vi "Property Finder (SubVI).vi"(8 "error in (no error)":errorcluster, 10 "Enum":enum16{"Read File", "Search for Property Name"}(ring), 11 "Property Name":string) -> (0 "error out":errorcluster, 3 "Property Value":string)   [LabVIEW 2018]
uses:
  <vilib>/regexp/Match Regular Expression.xnode
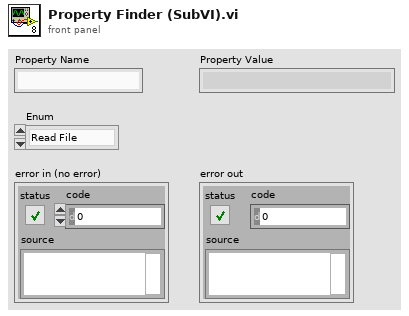
[diagram p1: front panel]
types:
  T1 = enum16{"open", "replace", "create", "open or create", "replace or create", "replace or create with confirmation"}
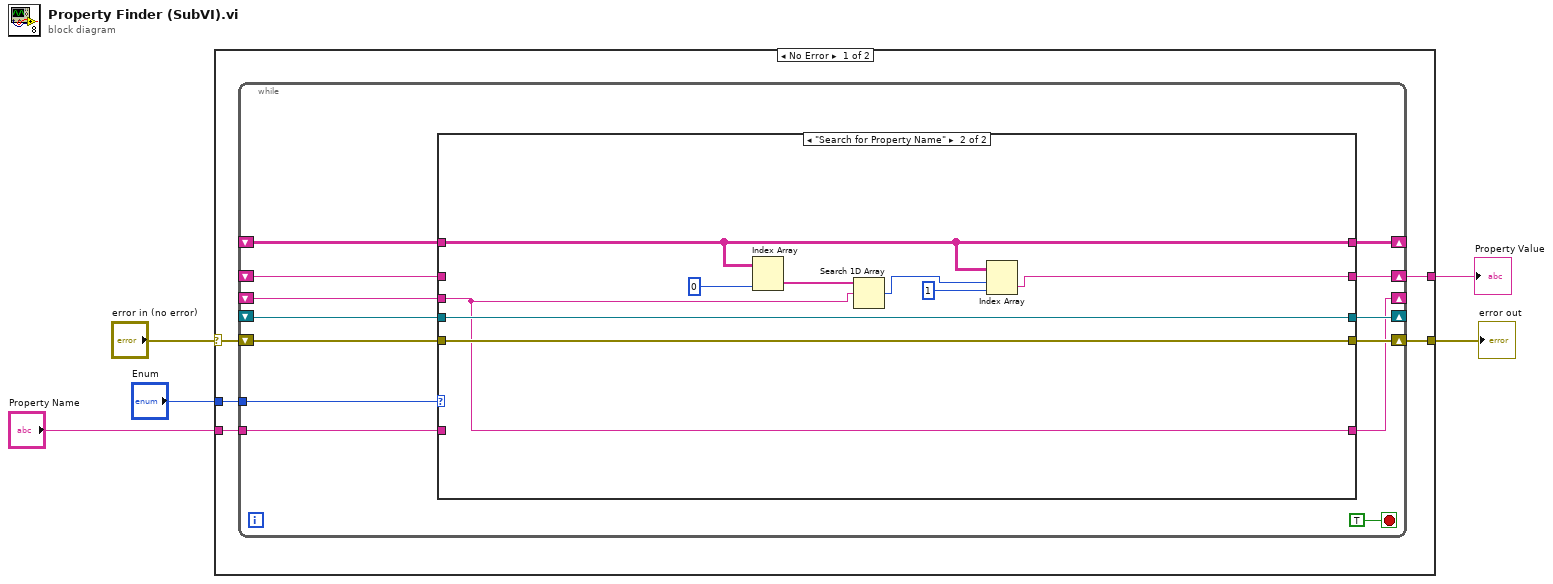
[diagram p0: block diagram]
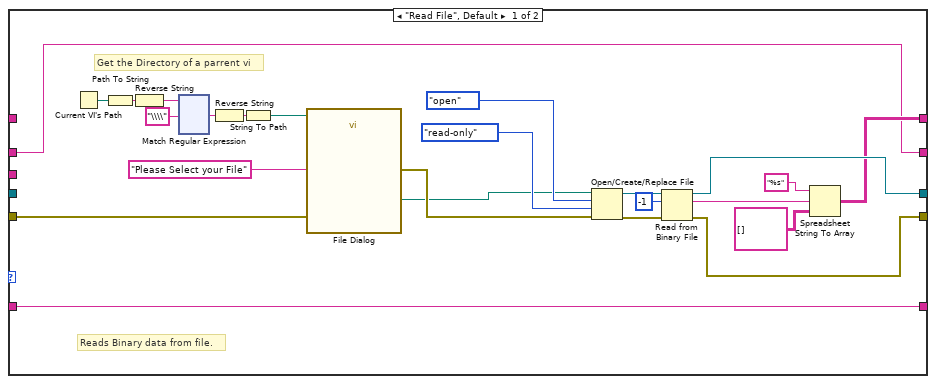
[diagram p2: hidden frame]
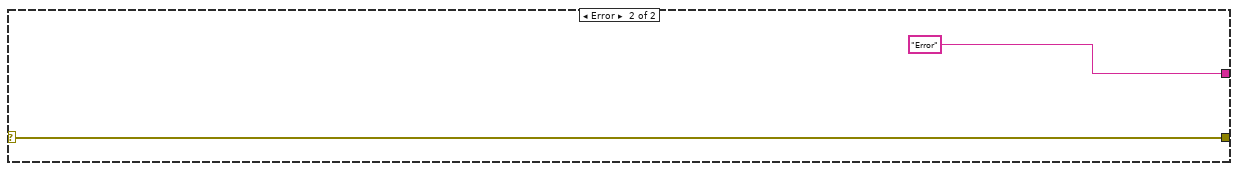
[diagram p3: hidden frame]
diagram:
  n1 = case shown="No Error" "error in (no error)" {
    selector: "error in (no error)" -> [w8 w172]
    tunnel: "Enum" -> [w10 _]
    tunnel: [w9 w172] -> w2
    tunnel: "Property Name" -> [w6 _]
    tunnel: [w7 "Error"] -> w5
    frame No Error {
      n2 = while {
        tunnel: w10 -> [w23]
        shift-right: [w21] -> w9
        shift-left: w8 -> [w20]
        shift-right: [w19] -> _
        shift-left: _ -> [w18]
        shift-right: [w16] -> _
        shift-left: _ -> [w17]
        shift-right: [w15] -> w7
        shift-left: _ -> [w14]
        shift-right: [w13] -> _
        shift-left: _ -> [w11]
        tunnel: w6 -> [w12]
        stop <- TRUE stop-if-true
        n3 = case shown="\"Search for Property Name\"" w23 {
          tunnel: [w28 w170] -> w21
          tunnel: w20 -> [w42 w170]
          tunnel: [w27 w169] -> w19
          tunnel: [w26 w166] -> w16
          tunnel: w18 -> [_ w169]
          tunnel: w17 -> [_ w166]
          tunnel: [w25 w163] -> w15
          tunnel: w14 -> [w25 _]
          tunnel: [w24 w162] -> w13
          tunnel: w12 -> [w24 _]
          tunnel: w11 -> [_ w162]
          frame "Read File", Default {
            # "Reads Binary data from file."
            # "Get the Directory of a parrent vi"
            n4 = Current VI's Path() -> (path=w34:path)
            n5 = Path To String(path=w34) -> (string=w35:string)
            n6 = Reverse String(1:w35) -> (0:w36:string)
            n7 = xnode "Match Regular Expression"("input string"=w36, "regular expression"="\\\\") -> ("after match"=w38:string)  [unwired: 4 in, 4 out]
            n8 = Reverse String(1:w38) -> (0:w39:string)
            n9 = String To Path(string=w39) -> (path=w33:path)
            n10 = call "File Dialog"("start path"=w33, "prompt"="Please Select your File", "error in"=w42) -> ("selected path"=w32:path, "error out"=w41:errorcluster)  [unwired: 9 in, 2 out]
            n11 = Open/Create/Replace File(file path (use dialog)=w32, error in=w41, operation (0:open)=T1."open", access (0:read/write)=enum16{"read/write", "read-only", "write-only"}."read-only") -> (refnum out=w45:refnum<file>, error out=w44:errorcluster)  [unwired: 2 in, 1 out]
            n12 = Read from Binary File(8:w44, 10:-1 ("count (1)"), 11:w45) -> (0:w28:errorcluster, 2:w29:string, 3:w27:refnum<file>)  [unwired: 3 in, 1 out]
            n13 = Spreadsheet String To Array(format string="%s", spreadsheet string=w29, array type (2D Dbl)=string[][] []) -> (array=w26:string[][])  [unwired: 1 in]
          }
          frame "Search for Property Name" {
            n14 = Index Array(array=w166, index (col)=0 ("disabled index (col)")) -> (element=w165:string[])  [unwired: 1 in]
            n15 = Search 1D Array(1D array=w165, element=w162) -> (index of element=w164:i32)  [unwired: 1 in]
            n16 = Index Array(array=w166, index (row)=w164, index (col)=1 ("disabled index (col)")) -> (element=w163:string)
          }
        }
      }
    }
    frame Error {
    }
  }
  "Property Value" <- w5
  "error out" <- w2
